vi "example_GArrayDownloadFile.vi"() -> ()   [LabVIEW 2020]
uses:
  <vilib>/Galil/resources/gclib/gclib.lvlib
  <vilib>/Galil/resources/gclibo/gclibo.lvlib
panel:
  in  "Command":string="LA"
  out "Response":string
  in  "File Location":string="C:\\Program Files (x86)\\Galil\\gclib\\examples\\labview\\array_download.csv"
  out "Error Out":errorcluster
  in  "IP Address":string="192.168.1.77"
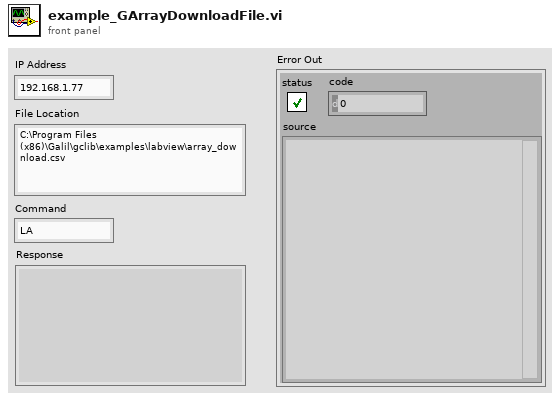
[diagram p1: front panel]
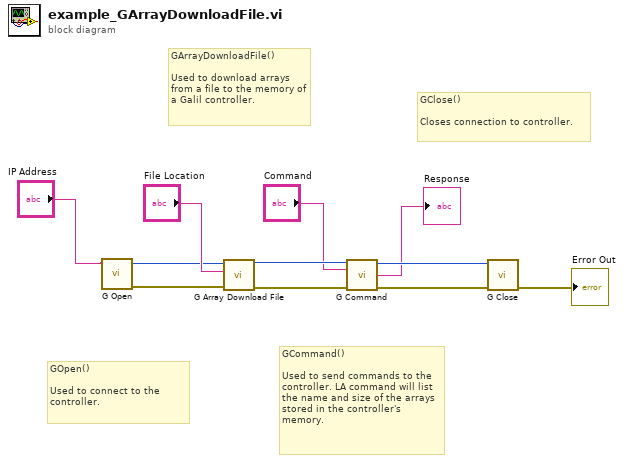
[diagram p0: block diagram]
diagram:
  # "GCommand()\n\nUsed to send commands to the controller. LA command will list the name and size of the arrays stored in the controller's memory."
  # "GArrayDownloadFile()\n\nUsed to download arrays from a file to the memory of a Galil controller."
  # "GClose()\n\nCloses connection to controller."
  # "GOpen()\n\nUsed to connect to the controller."
  n1 = call <vilib>:"G Open.vi"("address"="IP Address") -> ("error out"=w7:errorcluster, "g out"=w8:u64)  [unwired: 8 in]
  n2 = call <vilib>:"G Array Download File.vi"("error in (no error)"=w7, "file_path"="File Location", "g"=w8) -> ("error out"=w5:errorcluster, "g out"=w6:u64)  [unwired: 6 in]
  n3 = call <vilib>:"G Command.vi"("g"=w6, "command"="Command", "error in (no error)"=w5) -> ("g out"=w3:u64, "buffer out"=→"Response":string, "error out"=w4:errorcluster)  [unwired: 10 in]
  n4 = call <vilib>:"G Close.vi"("error in (no error)"=w4, "g"=w3) -> ("error out"=→"Error Out":errorcluster)  [unwired: 9 in]
